vi "DISP_ANN_STAT.vi"(0 "VISA IN":refnum<visa-resource-name>, 2 "Status Bar?":bool, 5 "error in":errorcluster) -> (14 "VISA Out":refnum<visa-resource-name>, 19 "error out":errorcluster)   [LabVIEW 2018, in "PNA-X.lvlib"]
doc: "DISPlay:ANNotation:STATus <ON | OFF> \n1587\n\n(Read-Write) Turns the status bar at the bottom of the screen ON or OFF. The status bar displays \ninformation for the active window. \nParameters \n<ON | OFF> ON (or 1) - turns status bar ON. \nOFF (or 0) - turns status bar OFF. \nExamples DISP:ANN:STAT ON \ndisplay:annotation:status off \nQuery Syntax DISPlay:ANNotation:STATus? \nReturn Type Boolean (1 = ON, 0 = OFF) \nDefault Last state that was set"
uses:
  PNA-X.lvlib
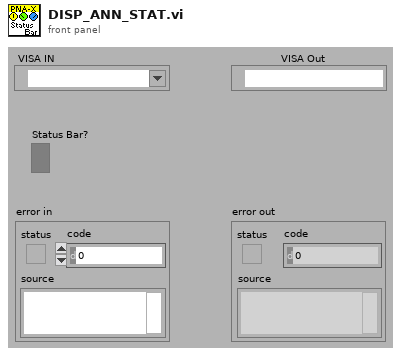
[diagram p1: front panel]
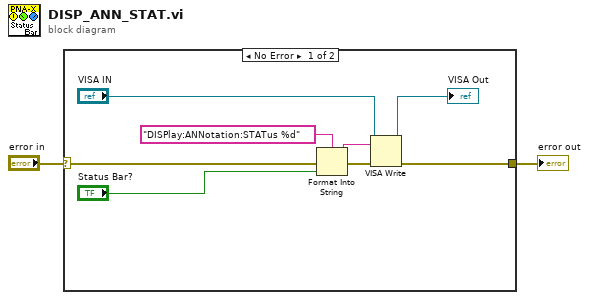
[diagram p0: block diagram]
diagram:
  n1 = case shown="No Error" "error in" {
    selector: "error in" -> [w10 w11]
    tunnel: [w5 w11] -> w1
    frame No Error {
      n2 = Format Into String(format string="DISPlay:ANNotation:STATus %d" ("Cmdline"), error in=w10, "Status Bar?") -> (resulting string=w8:string, error out=w9:errorcluster)  [unwired: 1 in]
      n3 = VISA Write(VISA resource name="VISA IN", write buffer=w8, error in (no error)=w9) -> (VISA resource name out=→"VISA Out":refnum<visa-resource-name>, error out=w5:errorcluster)  [unwired: 1 out]
    }
    frame Error {
    }
  }
  "error out" <- w1
